vi "Part 1.vi"(11 "Input":string) -> (3 "Output":i64)   [LabVIEW 2021]
uses:
  dc77b2c3-0248-4bfe-a632-ad9d94312f3f.vi
  <userlib>/_OpenG.lib/string/string.llb/Convert EOLs (String)__ogtk.vi
  <vilib>/Comparison/Equal/Equal Functor/Equal Functor.lvclass
panel:
  out "Map":string[][](array[string])
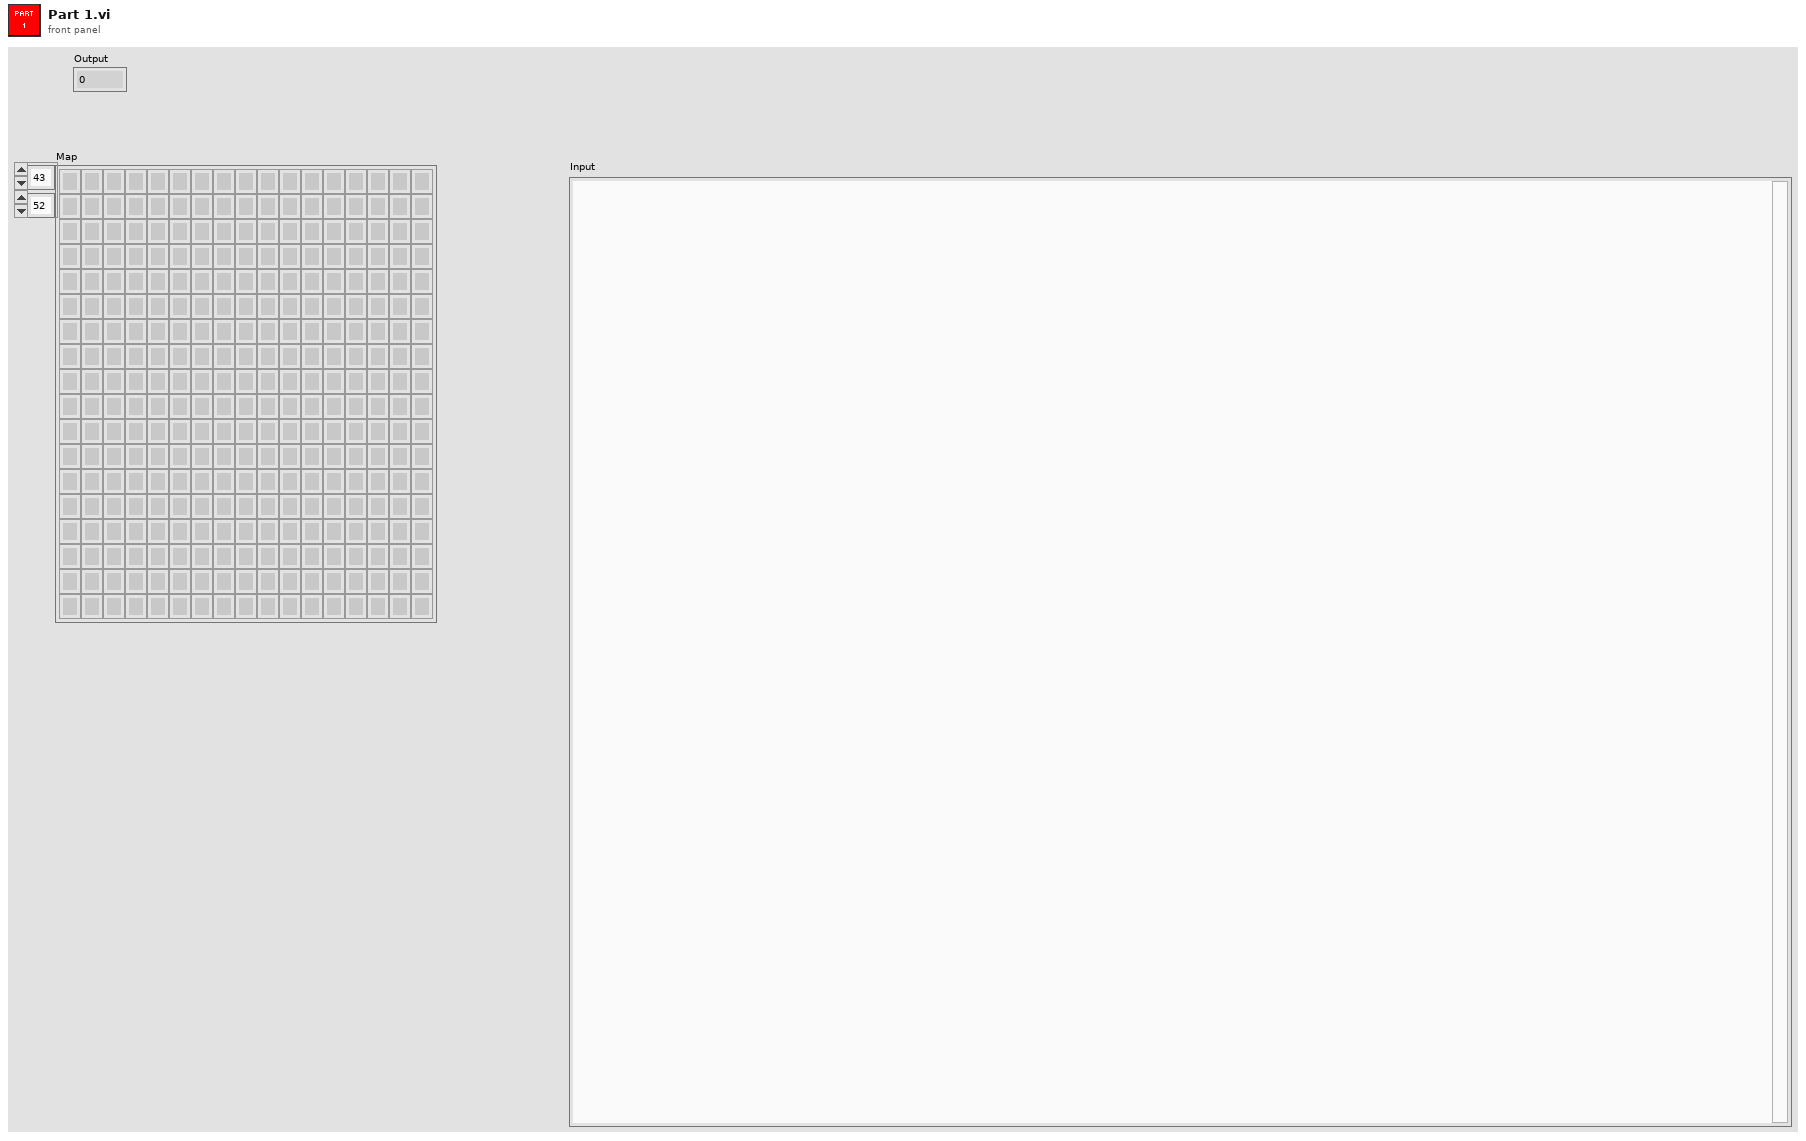
[diagram p1: front panel]
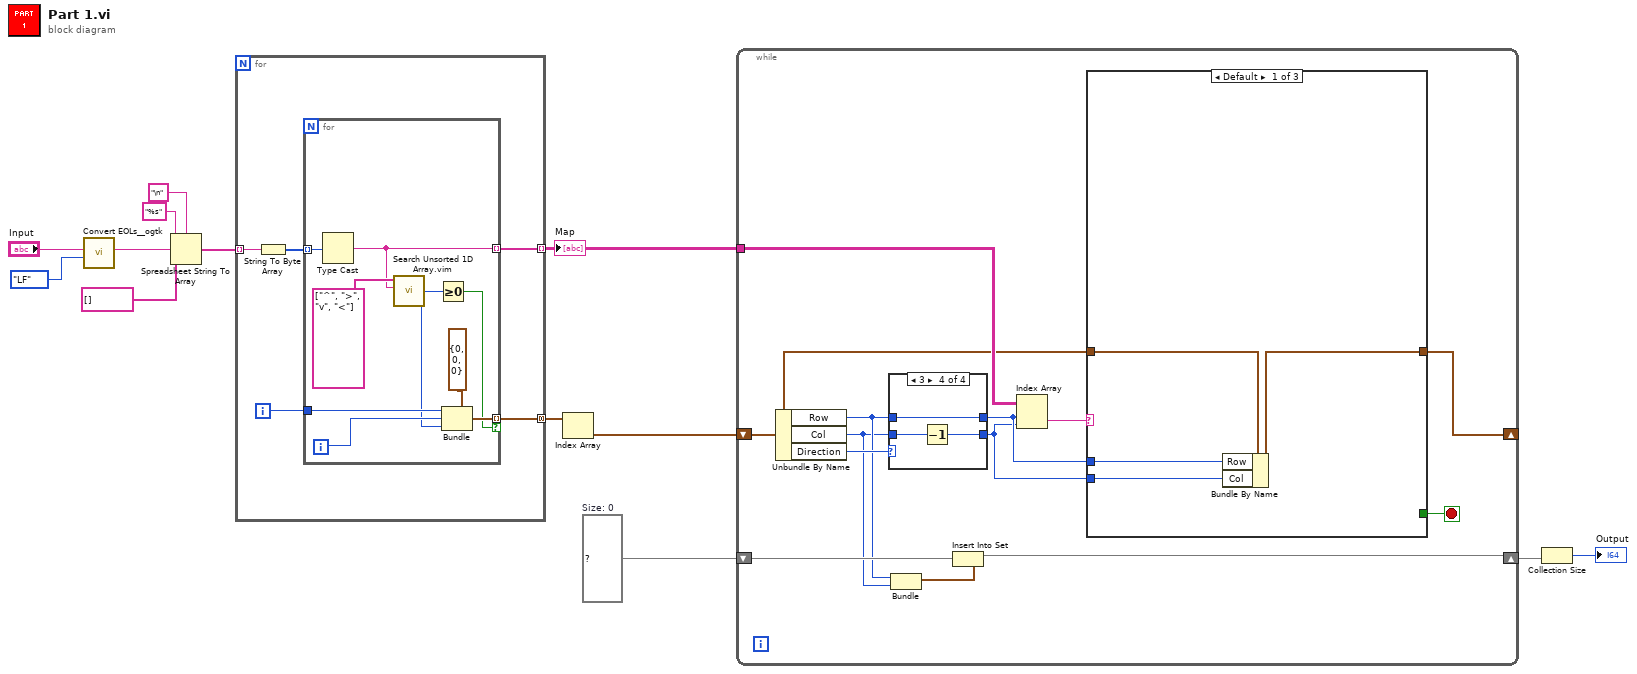
[diagram p0: block diagram]
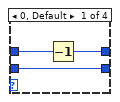
[diagram p2: hidden frame]
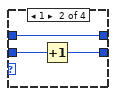
[diagram p3: hidden frame]
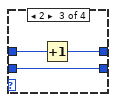
[diagram p4: hidden frame]
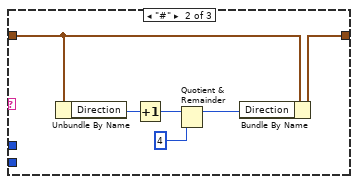
[diagram p5: hidden frame]
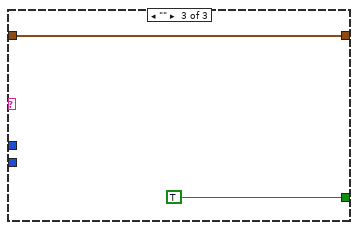
[diagram p6: hidden frame]
diagram:
  w4 = set{cluster{"Row":i32, "Col":i32}} {}  # Size: 0
  n1 = call-poly <userlib>:"Convert EOLs__ogtk.vi"("Convert to:"=enum16{"CR", "LF", "CRLF"}."LF", "String in"="Input") -> ("String out"=w9:string)  [unwired: 9 in]
  n2 = Spreadsheet String To Array(delimiter (Tab)="\n", format string="%s", spreadsheet string=w9, array type (2D Dbl)=string[] []) -> (array=w7:string[])
  n3 = for {
    tunnel: w7 -> [w18] mode=indexing
    tunnel: [w16] -> w1 mode=indexing
    tunnel: [w14] -> w6 mode=concatenating
    i -> [w15]
    n4 = String To Byte Array(string=w18) -> (unsigned byte array=w17:u8[])
    n5 = for {
      tunnel: w17 -> [w27] mode=indexing
      tunnel: [w20] -> w16 mode=indexing
      tunnel: w15 -> [w26]
      tunnel: [w22] -> w14 mode=indexing if=w21
      i -> [w25]
      n6 = Type Cast(x=w27) -> (*(type *) &x=w20:string)  [unwired: 1 in]
      n7 = call "Search Unsorted 1D Array.vim"("element"=w20, "unsorted 1D array"=string[] ["^", ">", "v", "<"]) -> ("index of element"=w23:i32)  [unwired: 9 in]
      n8 = Greater Or Equal To 0?(x=w23) -> (x >= 0?=w21:bool)
      n9 = Bundle(cluster=cluster{"Row":i32, "Col":i32, "Direction":i32} {"Row"=0, "Col"=0, "Direction"=0} ("Position"), "Row"=w26, "Col"=w25, "Direction"=w23) -> (w22:cluster{"Row":i32, "Col":i32, "Direction":i32})
    }
  }
  "Map" <- w1
  n10 = Index Array(array=w6) -> (element=w5:cluster{"Row":i32, "Col":i32, "Direction":i32})  [unwired: 1 in]
  n11 = while {
    shift-right: [w30] -> _
    shift-left: w5 -> [w31]
    shift-right: [w32] -> w3
    shift-left: w4 -> [w36]
    tunnel: w1 -> [w39]
    stop <- w37 stop-if-true
    n12 = Unbundle By Name(w31) -> ("Row"=w35:i32, "Col"=w34:i32, "Direction"=w40:i32)
    n13 = case shown="3" w40 {
      tunnel: w34 -> [w43 w46 w48 w52]
      tunnel: w35 -> [w42 w45 w49 w51]
      tunnel: [w43 w44 w48 w50] -> w28
      tunnel: [w41 w45 w47 w51] -> w29
      frame 0, Default {
        n14 = Decrement(x=w42) -> (x-1=w41:i32)
      }
      frame 1 {
        n15 = Increment(x=w46) -> (x+1=w44:i32)
      }
      frame 2 {
        n16 = Increment(x=w49) -> (x+1=w47:i32)
      }
      frame 3 {
        n17 = Decrement(x=w52) -> (x-1=w50:i32)
      }
    }
    n18 = Bundle("Row"=w35, "Col"=w34) -> (w33:cluster{"Row":i32, "Col":i32})  [unwired: 1 in]
    n19 = Insert Into Set(10:w33, 11:w36) -> (3:w32:set{cluster{"Row":i32, "Col":i32}})  [unwired: 1 out]
    n20 = Index Array(array=w39, index (row)=w29, index (col)=w28) -> (element=w38:string)
    n21 = case shown="Default" w38 {
      tunnel: [_ _ TRUE] -> w37
      tunnel: w31 -> [w56 w61 w63]
      tunnel: [w55 w62 w63] -> w30
      tunnel: w29 -> [w54 _ _]
      tunnel: w28 -> [w53 _ _]
      frame Default {
        n22 = Bundle By Name(cluster=w56, "Row"=w54, "Col"=w53) -> (w55:cluster{"Row":i32, "Col":i32, "Direction":i32})
      }
      frame "#" {
        n23 = Unbundle By Name(w61) -> ("Direction"=w60:i32)
        n24 = Increment(x=w60) -> (x+1=w59:i32)
        n25 = Quotient & Remainder(x=w59, y=4) -> (x-y*floor(x/y)=w58:i32)  [unwired: 1 out]
        n26 = Bundle By Name(cluster=w61, "Direction"=w58) -> (w62:cluster{"Row":i32, "Col":i32, "Direction":i32})
      }
      frame "" {
      }
    }
  }
  n27 = Collection Size(1:w3) -> (0:→"Output":i32)
